vi "Parse GID_DSA_Telemetry.vi"(10 "Data In":variant) -> (2 "GID_Status":T1 {"GID_2_DSA"."DSA_SS_0_2" format="%03b"; "GID_2_DSA"."DSA_Word_2_Sent" format="%04x"; "GID_2_DSA"."SSA1_0_2" format="%03b"; "GID_2_DSA"."DSA_SS_0_2_BTE" format="%03b"; "GID_2_DSA"."SSA2_0_2" format="%03b"; "GID_1_DSA"."DSA_SS_0_2" format="%03b"; "GID_1_DSA"."DSA_Word_2_Sent" format="%04x"; "GID_1_DSA"."SSA1_0_2" format="%03b"; "GID_1_DSA"."DSA_SS_0_2_BTE" format="%03b"; "GID_1_DSA"."SSA2_0_2" format="%03b"})   [LabVIEW 2019]
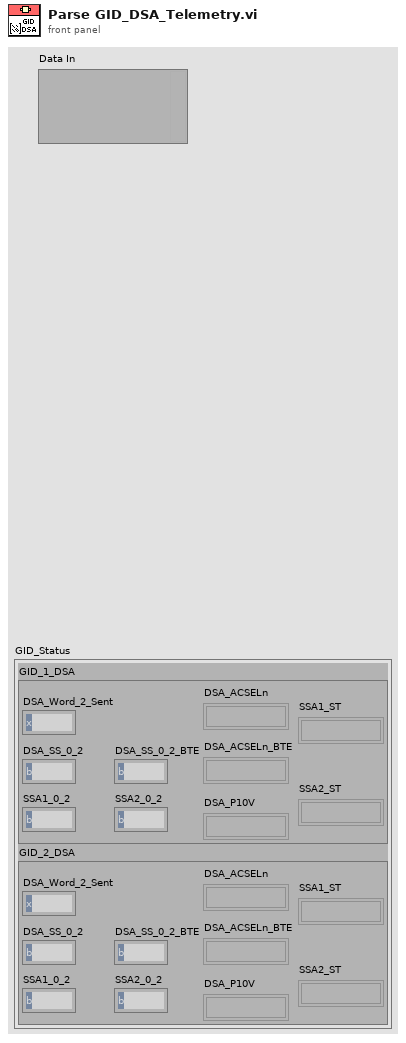
[diagram p1: front panel]
types:
  T1 = cluster{"GID_1_DSA":cluster{"DSA_Word_2_Sent":u16, "DSA_SS_0_2":u8, "DSA_SS_0_2_BTE":u8, "SSA1_0_2":u8, "SSA2_0_2":u8, "DSA_ACSELn":bool, "DSA_ACSELn_BTE":bool, "DSA_P10V":bool, "SSA1_ST":bool, "SSA2_ST":bool}, "GID_2_DSA":cluster{"DSA_Word_2_Sent":u16, "DSA_SS_0_2":u8, "DSA_SS_0_2_BTE":u8, "SSA1_0_2":u8, "SSA2_0_2":u8, "DSA_ACSELn":bool, "DSA_ACSELn_BTE":bool, "DSA_P10V":bool, "SSA1_ST":bool, "SSA2_ST":bool}}
  T2 = cluster{"GID_1_DSA":cluster{"DSA_Word_2_Sent":u16, "DSA_SS_0_2":u8, "DSA_SS_0_2__BTE":u8, "SSA1_0_2":u8, "SSA2_0_2":u8, "DSA_ACSELn":bool, "DSA_ACSELn_BTE":bool, "DSA_P10V":bool, "SSA1_ST":bool, "SSA2_ST":bool}, "GID_2_DSA":cluster{"DSA_Word_2_Sent":u16, "DSA_SS_0_2":u8, "DSA_SS_0_2__BTE":u8, "SSA1_0_2":u8, "SSA2_0_2":u8, "DSA_ACSELn":bool, "DSA_ACSELn_BTE":bool, "DSA_P10V":bool, "SSA1_ST":bool, "SSA2_ST":bool}}
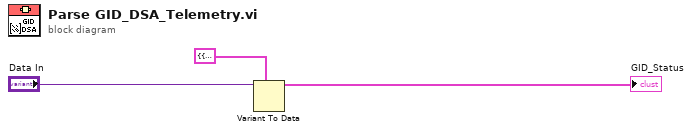
[diagram p0: block diagram]
diagram:
  n1 = Variant To Data(type=T2 {"GID_1_DSA"={"DSA_Word_2_Sent"=0, "DSA_SS_0_2"=0, "DSA_SS_0_2__BTE"=0, "SSA1_0_2"=0, "SSA2_0_2"=0, "DSA_ACSELn"=FALSE, "DSA_ACSELn_BTE"=FALSE, "DSA_P10V"=FALSE, "SSA1_ST"=FALSE, "SSA2_ST"=FALSE}, "GID_2_DSA"={"DSA_Word_2_Sent"=0, "DSA_SS_0_2"=0, "DSA_SS_0_2__BTE"=0, "SSA1_0_2"=0, "SSA2_0_2"=0, "DSA_ACSELn"=FALSE, "DSA_ACSELn_BTE"=FALSE, "DSA_P10V"=FALSE, "SSA1_ST"=FALSE, "SSA2_ST"=FALSE}} ("data"), Variant="Data In") -> (data=→"GID_Status":T2)  [unwired: 1 in, 1 out]
